vi "String.Check if Str Array Items are in a Str Array List.vi"(8 "error in (no error)":errorcluster, 9 "Case Sensitive":bool, 10 "Items to Check":string[](array[string]), 11 "List":string[](array[string])) -> (0 "error out":errorcluster, 2 "All Items in list":bool, 3 "Items Not in List":string[](array[string]))   [LabVIEW 2019]
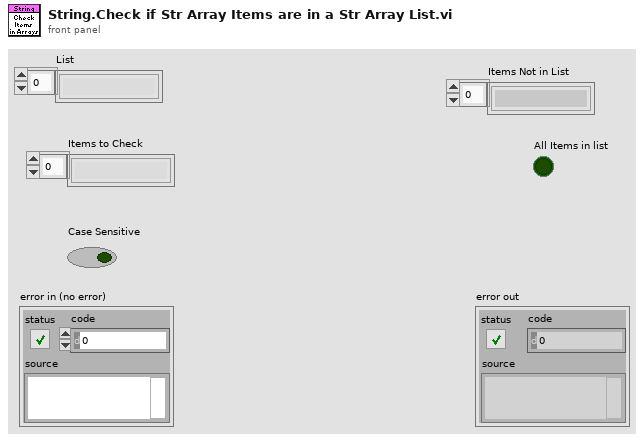
[diagram p1: front panel]
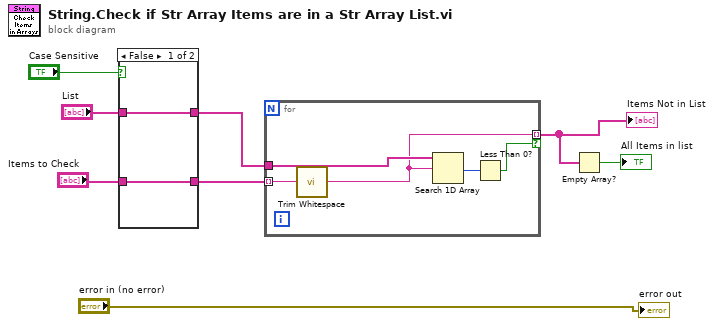
[diagram p0: block diagram]
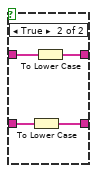
[diagram p2: hidden frame]
diagram:
  n1 = case shown="False" "Case Sensitive" {
    tunnel: "List" -> [w10 w14]
    tunnel: [w10 w13] -> w3
    tunnel: "Items to Check" -> [w9 w12]
    tunnel: [w9 w11] -> w1
    frame False {
    }
    frame True {
      n2 = To Lower Case(string=w12) -> (all lower case string=w11:string[])
      n3 = To Lower Case(string=w14) -> (all lower case string=w13:string[])
    }
  }
  n4 = for {
    tunnel: w1 -> [w19] mode=indexing
    tunnel: w3 -> [w16]
    tunnel: [w15] -> w7 mode=indexing if=w17
    n5 = call <vilib>:"Trim Whitespace.vi"("string"=w19) -> ("trimmed string"=w15:string)  [unwired: 1 in]
    n6 = Search 1D Array(1D array=w16, element=w15) -> (index of element=w18:i32)  [unwired: 1 in]
    n7 = Less Than 0?(x=w18) -> (x < 0?=w17:bool)
  }
  "Items Not in List" <- w7
  n8 = Empty Array?(array=w7) -> (empty?=→"All Items in list":bool)
  "error out" <- "error in (no error)"
